vi "localArquivo.vi"(7 "quantidadeDeArquivos":i16, 8 "numeroDoArquivo":i16, 9 "extensão":string, 10 "Nome do arquivo":string, 11 "Local":path) -> (3 "Path":path)   [LabVIEW 2012]
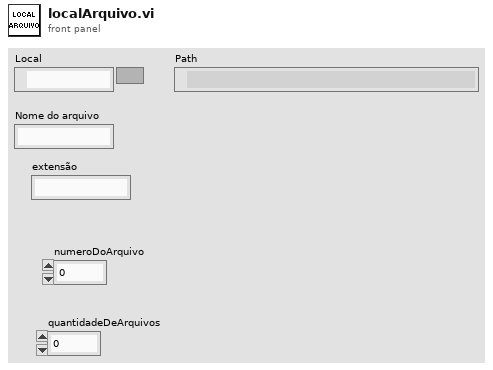
[diagram p1: front panel]
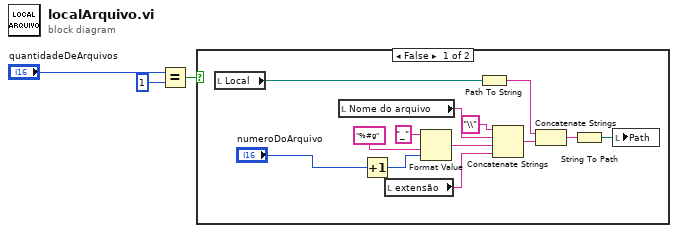
[diagram p0: block diagram]
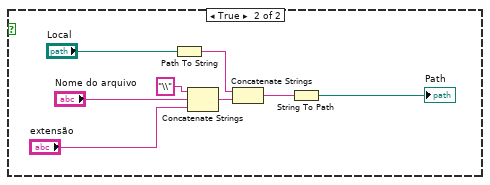
[diagram p2: hidden frame]
diagram:
  n1 = Equal?(x="quantidadeDeArquivos", y=i64 1) -> (x = y?=w2:bool)
  n2 = case shown="False" w2 {
    frame False {
      n3 = local read "Local"() -> (w13:path)
      n4 = local read "Nome do arquivo"() -> (w12:string)
      n5 = Increment(x="numeroDoArquivo") -> (x+1=w8:i16)
      n6 = local read "extensão"() -> (w10:string)
      n7 = Format Value(string ("")="_", format string="%#g", value (0)=w8) -> (output string=w7:string)
      n8 = Path To String(path=w13) -> (string=w15:string)
      n9 = Concatenate Strings("\\" ("string"), w12, w7, w10) -> (w16:string)
      n10 = Concatenate Strings(w15, w16) -> (w14:string)
      n11 = String To Path(string=w14) -> (path=w6:path)
      n12 = local write "Path"(w6) -> ()
    }
    frame True {
      n13 = Path To String(path="Local") -> (string=w22:string)
      n14 = Concatenate Strings("\\", "Nome do arquivo", "extensão") -> (w23:string)
      n15 = Concatenate Strings(w22, w23) -> (w21:string)
      n16 = String To Path(string=w21) -> (path=→"Path":path)
    }
  }
